vi "StringToU64(cast).vi"(1 "String":string) -> (0 "U64":u64)   [LabVIEW 2012]
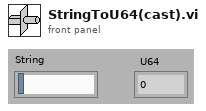
[diagram p1: front panel]
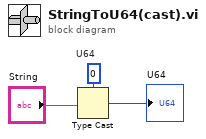
[diagram p0: block diagram]
diagram:
  w2 = u64 0  # U64
  n1 = Type Cast(type=w2, x="String") -> (*(type *) &x=→"U64":u64)
